vi "Z Go.vi"(6 "Return Immediately":bool, 8 "error in (no error)":errorcluster, 9 "Speed In":dbl format="%#_13g", 10 "Position In":dbl format="%#_13g", 11 "Gantry In":refnum<k24>) -> (0 "error out":errorcluster, 1 "Speed Out":dbl, 2 "Position Out":dbl, 3 "Gantry Out":refnum<k24>)   [LabVIEW 2020, in "Motion.lvclass"]
uses:
  Motion.lvclass
  C:/Program Files (x86)/Aerotech/A3200/LabVIEW/2010/Bin/Aerotech.A3200.dll
  Program Files (x86)/Aerotech/A3200/LabVIEW/2010/Bin/Aerotech.A3200.dll
  Motion.lvclass/Motion.ctl
  Drivers/Aerotech A3200/Aerotech.lvlib
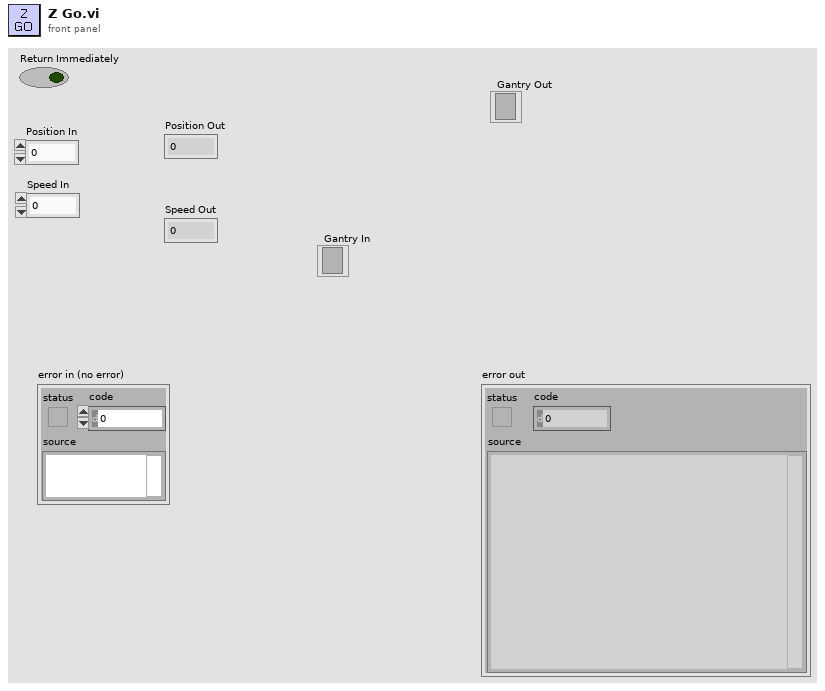
[diagram p1: front panel]
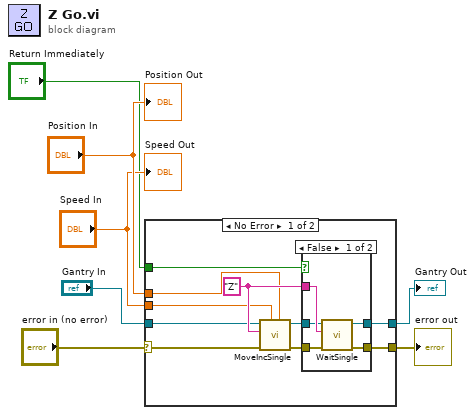
[diagram p0: block diagram]
diagram:
  n1 = case shown="No Error" "error in (no error)" {
    selector: "error in (no error)" -> [w9 w26]
    tunnel: [w8 w26] -> w6
    tunnel: "Gantry In" -> [w16 w25]
    tunnel: [w14 w25] -> w4
    tunnel: "Position In" -> [w13 _]
    tunnel: "Speed In" -> [w12 _]
    tunnel: "Return Immediately" -> [w11 _]
    frame No Error {
      w17 = "Z"
      n2 = call "MoveIncSingle.vi"("distance"=w13, "speed"=w12, "error in (no error)"=w9, "axis name"=w17, "controller in"=w16) -> ("error out"=w10:errorcluster, "controller out"=w15:refnum<k24>)  [unwired: 5 in]
      n3 = case shown="False" w11 {
        tunnel: w17 -> [w22 _]
        tunnel: w15 -> [w21 w24]
        tunnel: [w20 w24] -> w14
        tunnel: w10 -> [w19 w23]
        tunnel: [w18 w23] -> w8
        frame False {
          n4 = call "WaitSingle.vi"("error in (no error)"=w19, "axis name"=w22, "controller in"=w21) -> ("error out"=w18:errorcluster, "controller out"=w20:refnum<k24>)  [unwired: 6 in, 1 out]
        }
        frame True {
        }
      }
    }
    frame Error {
    }
  }
  "error out" <- w6
  "Gantry Out" <- w4
  "Speed Out" <- "Speed In"
  "Position Out" <- "Position In"
